vi "Read HDF5.vi"(8 "error in (no error)":errorcluster, 10 "path":path, 11 "LV to ITX.lvclass":refnum<class "LV to ITX.lvclass">) -> (0 "error out":errorcluster, 2 "Array":T1[](array[typedef]), 3 "LV to ITX.lvclass":refnum<class "LV to ITX.lvclass">, 4 "Comments":string, 6 "Igor Commands":string)   [LabVIEW 2016, in "LV to ITX.lvclass"]
uses:
  LV to ITX.lvclass
  Typedefs/Dictionary--cluster.ctl
  <vilib>/addons/h5labview2/file/H5Fmode.ctl
  LV to ITX.lvclass/LV to ITX.ctl
  <vilib>/addons/h5labview2/base/lib_path.vi
  <vilib>/addons/h5labview2/base/H5Equery.vi
  <vilib>/addons/h5labview2/dataset/H5Dread.llb/H5Dread.xnode
  <vilib>/addons/h5labview2/file/H5F.lvlib
  <vilib>/addons/h5labview2/group/H5G.lvlib
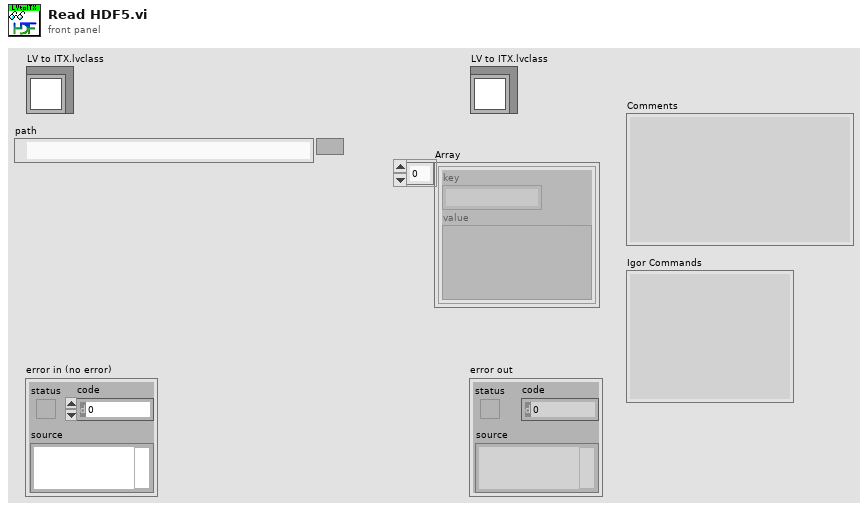
[diagram p1: front panel]
types:
  T1 = typedef "LV to ITX.lvclass/Dictionary--cluster.ctl" = cluster{"key":string, "value":variant}
  T2 = typedef "H5F.lvlib/H5Fmode.ctl" = enum16{"read-only", "read-write", "overwrite", "create new", "open or create"}
  T3 = typedef "hid_t.ctl" = i32
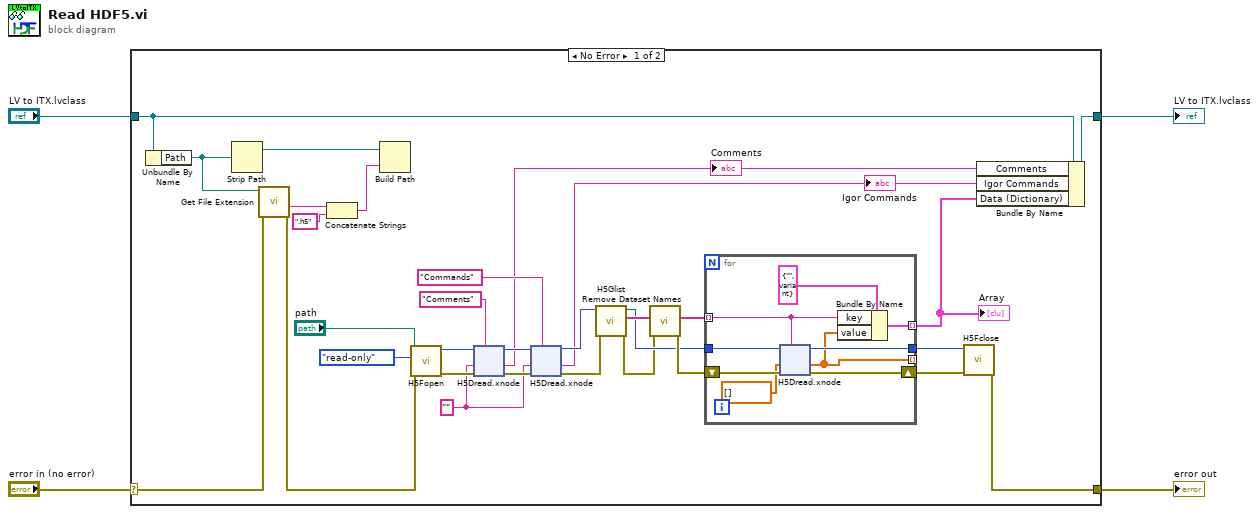
[diagram p0: block diagram]
diagram:
  n1 = case shown="No Error" "error in (no error)" {
    selector: "error in (no error)" -> [w19 w90]
    tunnel: [w24 w90] -> w1
    tunnel: [w20 w91] -> w2
    tunnel: "LV to ITX.lvclass" -> [w21 w91]
    frame No Error {
      w9 = "" ("attrib name")
      n2 = Unbundle By Name(w21) -> ("Path"=w23:path)
      n3 = Strip Path(path=w23) -> (stripped path=w32:path)  [unwired: 1 out]
      n4 = call <vilib>:"Get File Extension.vi"("error in (no error)"=w19, "file"=w23) -> ("error out"=w30:errorcluster, "filename without extension"=w34:string)  [unwired: 5 in, 3 out]
      n5 = Concatenate Strings(w34, ".h5" ("string")) -> (w31:string)
      n6 = Build Path(base path=w32, name or relative path=w31) -> ()  [unwired: 1 out]
      n7 = call <vilib>:"H5Fopen.vi"("error in (no error)"=w30, "mode (read-only)"=H5Fmode."read-only" ("mode"), "path"="path") -> ("error out"=w29:errorcluster, "ref out"=w22:T3)  [unwired: 7 in]
      n8 = xnode "H5Dread.xnode"("dataset name (this)"="Comments" ("attrib name"), "error in (no error)"=w29, "default"=w9, "ref in"=w22) -> ("error out"=w27:errorcluster, "data"=w16:string, "ref out"=w26:i32)  [unwired: 2 in, 1 out]
      "Comments" <- w16
      n9 = xnode "H5Dread.xnode"("dataset name (this)"="Commands" ("attrib name"), "error in (no error)"=w27, "default"=w9, "ref in"=w26) -> ("error out"=w7:errorcluster, "data"=w17:string, "ref out"=w18:i32)  [unwired: 2 in, 1 out]
      "Igor Commands" <- w17
      n10 = call <vilib>:"H5Glist.vi"("error in (no error)"=w7, "ref in"=w18) -> ("error out"=w6:errorcluster, "names"=w12:string[], "ref out"=w10:T3)  [unwired: 6 in, 1 out]
      n11 = call "Remove Dataset Names.vi"("error in (no error)"=w6, "Dataset Names"=w12) -> ("error out"=w11:errorcluster, "Name less Commands and Comments"=w8:string[])  [unwired: 8 in]
      n12 = for {
        shift-right: [w44] -> w14
        shift-left: w11 -> [w43]
        tunnel: w10 -> [w42]
        tunnel: [w41] -> w13
        tunnel: w8 -> [w37] mode=indexing
        tunnel: [w38] -> _ mode=indexing
        tunnel: [w36] -> w5 mode=indexing
        n13 = xnode "H5Dread.xnode"("dataset name (this)"=w37, "error in (no error)"=w43, "default"=dbl[] [] ("array type (2D Dbl)"), "ref in"=w42) -> ("error out"=w44:errorcluster, "data"=w38:dbl[], "ref out"=w41:i32)  [unwired: 2 in, 1 out]
        n14 = Bundle By Name(cluster=T1 {"key"="", "value"=variant} ("key-value"), "key"=w37, "value"=w38) -> (w36:T1)
      }
      "Array" <- w5
      n15 = call <vilib>:"H5Fclose.vi"("error in (no error)"=w14, "ref"=w13) -> ("error out"=w24:errorcluster)  [unwired: 9 in]
      n16 = Bundle By Name(cluster=w21, "Comments"=w16, "Igor Commands"=w17, "Data (Dictionary)"=w5) -> (w20:refnum<class "LV to ITX.lvclass">)
    }
    frame Error {
    }
  }
  "error out" <- w1
  "LV to ITX.lvclass" <- w2
